vi "Rectangular Target - 2013.vi"() -> ()   [LabVIEW 2012]
doc: "This VI demonstrates how to do target processing on a laptop computer. It uses the same MJPG VI as the dashboard, sets a few of the important camera properties that impact processing, and carries out the same processing steps as the RT example also included in this project."
uses:
  <vilib>/Rock Robotics/WPI/Camera/WPI_CameraImageSize.ctl
  <vilib>/Rock Robotics/WPI/Camera/WPI_CameraWhite Balance Values.ctl
  <vilib>/vision/NI_Vision_Development_Module.lvlib
panel:
  in  "Camera Type":enum16{"206", "1011"}(ring)=enum."1011"
  in  "Image Source":enum32{"File Images", "Live Camera"}(tab)
  in  "Directory":path
  in  "File List":i32(listbox)
  in  "Camera IP Address":string="192.168.0.90"
  in  "Camera Settings":T2={"FPS"=30, "Compression"=30, "Image Size"=enum."320x240"}
  out "Target Info":T3(array[cluster])
  in  "Area Size Limit %":dbl=0.5
  in  "Particle Count Limit":i32=10
  in  "Score Limits":T4={"Rect Coverage"=60.0, "X Edge Strength"=40.0, "Y Edge Strength"=60.0, "Center"=75.0, "Outer"=75.0}
  in  "Processing":enum32{"Color", "Monochrome"}(tab)
  out "Value":cluster{i32, i32}
  out "Saturation":cluster{i32, i32}
  in  "Value":i32=255
  in  "Saturation":i32=255
  in  "Hue":i32(knob)=65 scale=0.0..255.0
  in  "Margins":cluster{"Hue":i32, "Sat":i32, "Val":i32}={"Hue"=33, "Sat"=53, "Val"=9} {"Sat" scale=0.0..80.0; "Val" scale=0.0..80.0; "Hue" scale=0.0..80.0}
  out "Hue":cluster{i32, i32}
  in  "Range":cluster{"Lower value":sgl, "Upper value":sgl}={"Lower value"=150.0, "Upper value"=255.0} {"Lower value" scale=0.0..255.0; "Upper value" scale=0.0..255.0}
  in  "Color Plane":i32(ring)=6 items=["Red", "Green", "Blue", "Hue", "Saturation", "Luminance", "Value", "Intensity"]
  in  "Annotate":bool=TRUE
  out "Processed Image":T5(plugin-control)
  out "Original Image":T5(plugin-control)
  # "Information:\nProcessing can be based on color or light intensity.\nParticles within the image are scored by rectangle coverage, aspect ratio, and\nedge strength/hollowness. A particle is considered a target if all scores\nare above the score limits you set. Particles can be annotated -- surrounded by\na rectangle and scores drawn to the left .\nTo control the number of particles being scored, use the count limit and the size\nlimit.\nBe sure to set the Camera IP before running. The distance calculation uses the\ncamera type to index the value of the lens view angle."
  # "Click in the image to choose  color for processing."
  # "Green scores are above the limit, orange are below. Inner/outer rect\nindicates all passed."
  # "Set before running."
  # "Lower/Upper"
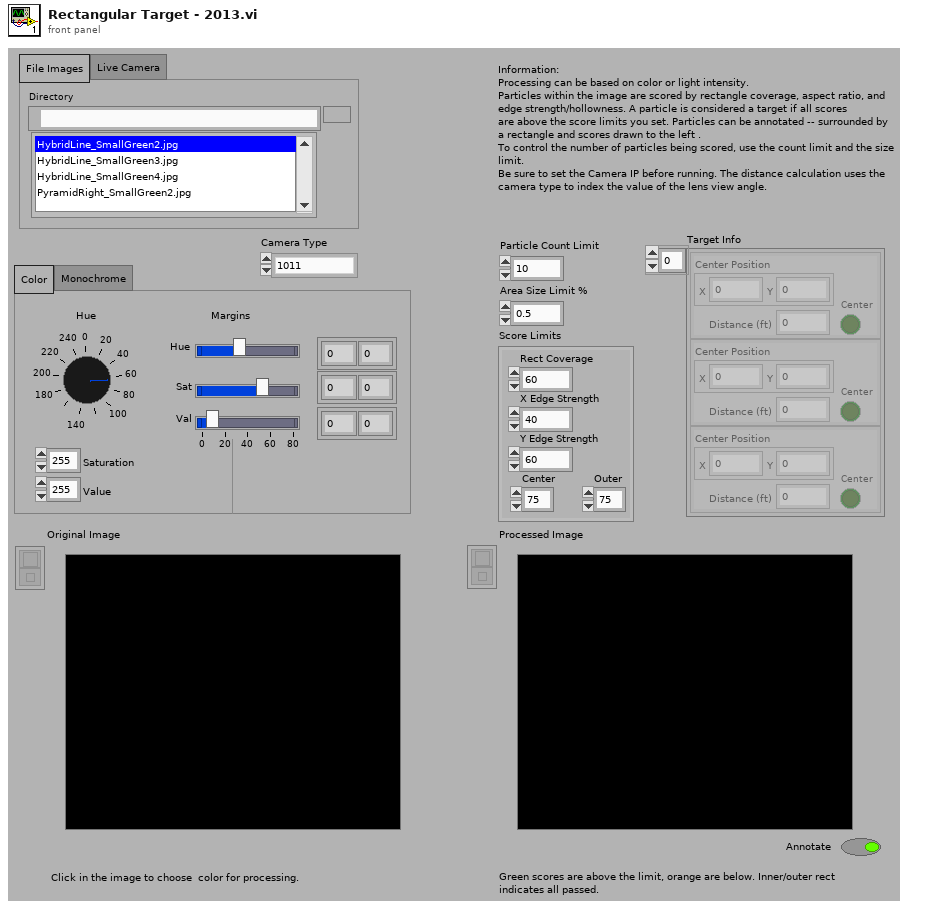
[diagram p1: front panel]
types:
  T1 = typedef "WPI_CameraImageSize.ctl" = enum16{"640x480", "320x240", "160x120"}
  T2 = cluster{"FPS":i32, "Compression":i32, "Image Size":T1}
  T3 = cluster{"Center Position":cluster{"X":dbl, "Y":dbl}, "Distance (ft)":dbl, "Center":bool}[]
  T4 = cluster{"Rect Coverage":dbl, "X Edge Strength":dbl, "Y Edge Strength":dbl, "Center":dbl, "Outer":dbl}
  T5 = typedef "IMAQ Image.ctl" = refnum<image>
  T6 = typedef "WPI_CameraWhite Balance Values.ctl" = enum16{"Auto", "Fixed indoor", "Fixed outdoor 1", "Fixed outdoor 2", "Fixed fluorescent 1", "Fixed fluorescent 2", "Hold current"}
  T7 = typedef "Image Type" = u32
  T8 = typedef "WPI_CameraDevRef.ctl" = cluster{"Camera Address":string, "CameraStatus":errorcluster, "Acquire Image Notifier":refnum<notifier>}
  T9 = cluster{"Position":cluster{"X":dbl, "Y":dbl}, "Distance (ft)":dbl, bool}[]
  T10 = cluster{cluster{"Left":dbl, "Top":dbl, "Right":dbl, "Bottom":dbl}, "Scores":dbl[], cluster{"Long":dbl, "Short":dbl}}[]
  T11 = cluster{"Target Center (-1 to 1)":cluster{"X":dbl, "Y":dbl}, "Distance (ft)":dbl, "Center Target":bool}
  T12 = cluster{"Target Center (-1 to 1)":cluster{"X":dbl, "Y":dbl}, "Distance (ft)":dbl, "Center Target":bool}[]
  T13 = cluster{"Left":dbl, "Top":dbl, "Right":dbl, "Bottom":dbl}
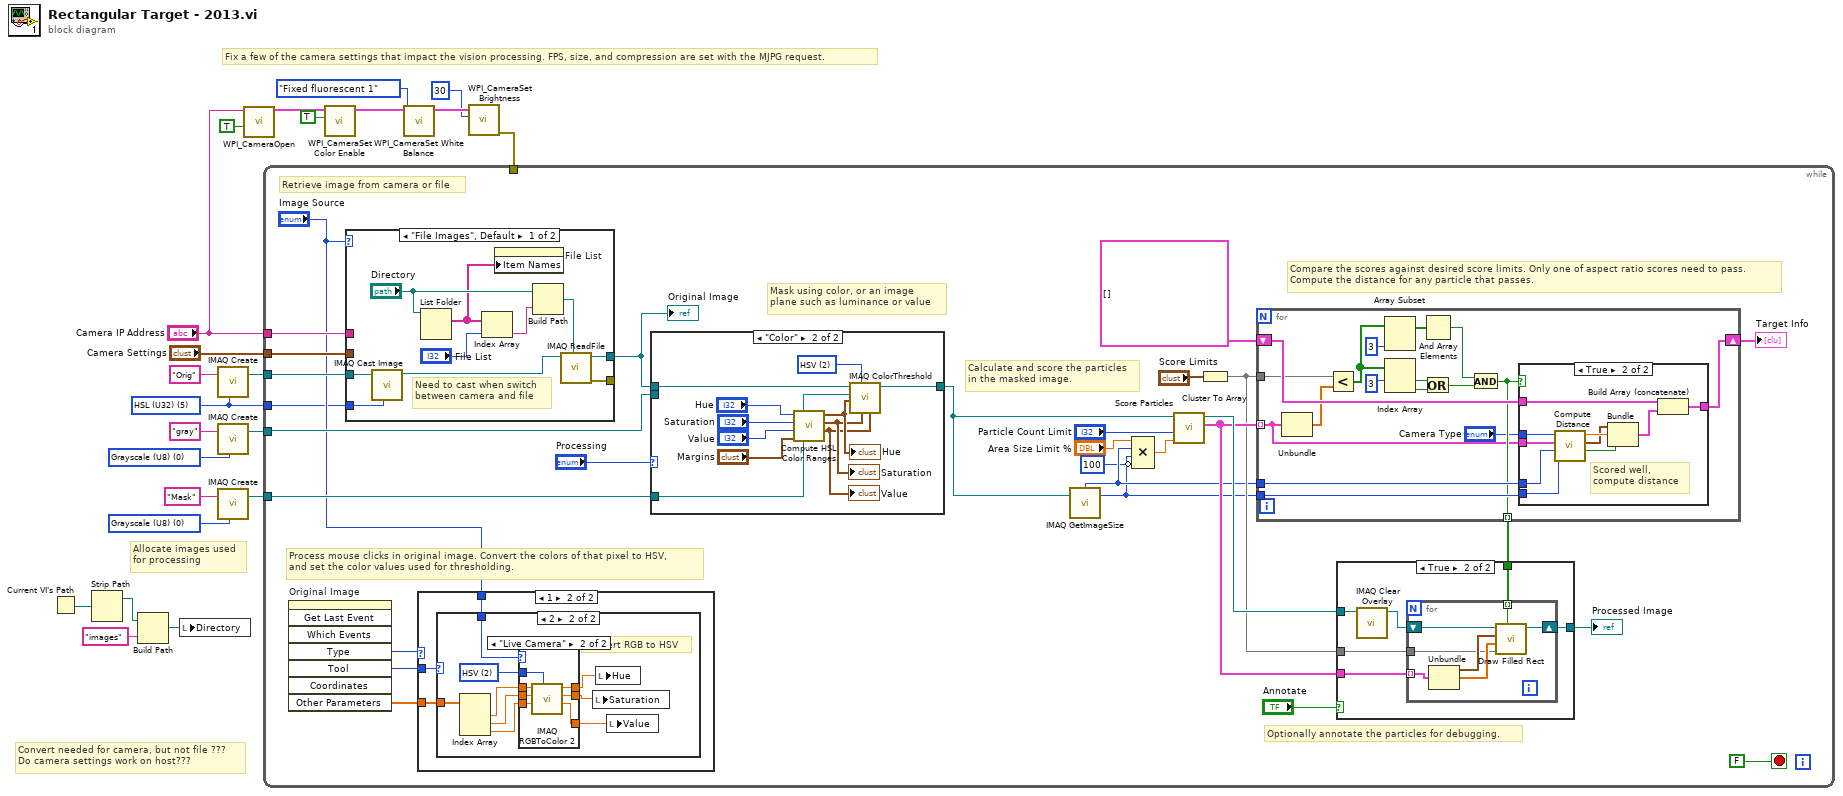
[diagram p0: block diagram]
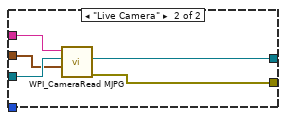
[diagram p2: hidden frame]
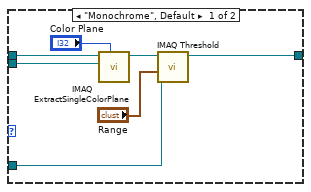
[diagram p4: hidden frame]
diagram:
  w17 = T7 0 items=["Grayscale (U8)", "Grayscale (I16)", "Grayscale (SGL)", "Complex (CSG)", "RGB (U32)", "HSL (U32)", "RGB (U64)", "Grayscale (U16)"] ("Image Type")
  w1 = T7 5 items=["Grayscale (U8)", "Grayscale (I16)", "Grayscale (SGL)", "Complex (CSG)", "RGB (U32)", "HSL (U32)", "RGB (U64)", "Grayscale (U16)"] ("Image Type")
  w23 = T7 0 items=["Grayscale (U8)", "Grayscale (I16)", "Grayscale (SGL)", "Complex (CSG)", "RGB (U32)", "HSL (U32)", "RGB (U64)", "Grayscale (U16)"] ("Image Type")
  # "Convert needed for camera, but not file ???\nDo camera settings work on host???"
  # "Allocate images used\nfor processing"
  # "Fix a few of the camera settings that impact the vision processing. FPS, size, and compression are set with the MJPG request."
  n1 = Current VI's Path() -> (path=w5:path)
  n2 = Strip Path(path=w5) -> (stripped path=w3:path)  [unwired: 1 out]
  n3 = Build Path(base path=w3, name or relative path="images") -> (appended path=w2:path)
  n4 = local write "Directory"(w2) -> ()
  n5 = call "IMAQ Create"("Image Name"="Orig", "Image Type"=w1) -> ("New Image"=w20:T5)  [unwired: 2 in, 2 out]
  n6 = call "IMAQ Create"("Image Name"="gray", "Image Type"=w23) -> ("New Image"=w19:T5)  [unwired: 2 in, 2 out]
  n7 = call "IMAQ Create"("Image Name"="Mask", "Image Type"=w17) -> ("New Image"=w16:T5)  [unwired: 2 in, 2 out]
  n8 = call <vilib>:"WPI_CameraOpen.vi"("Disallow Simulation"=TRUE, "Camera Address"="Camera IP Address") -> ("CameraDevRef"=w12:T8)  [unwired: 8 in, 1 out]
  n9 = call <vilib>:"WPI_CameraSet Color Enable.vi"("Color Enabled"=TRUE, "CameraDevRef"=w12) -> ("CameraDevRef Out"=w10:T8)  [unwired: 8 in, 1 out]
  n10 = call <vilib>:"WPI_CameraSet White Balance.vi"("White Balance"=WPI_CameraWhite_Balance_Values."Fixed fluorescent 1", "CameraDevRef"=w10) -> ("CameraDevRef Out"=w8:T8)  [unwired: 8 in, 1 out]
  n11 = call <vilib>:"WPI_CameraSet Brightness.vi"("Brightness"=30, "CameraDevRef"=w8) -> ("error out"=w14:errorcluster)  [unwired: 8 in, 1 out]
  n12 = while {
    tunnel: w20 -> [w45]
    tunnel: w19 -> [w52]
    tunnel: w16 -> [w31]
    tunnel: "Camera IP Address" -> [w43]
    tunnel: w14 -> [_]
    tunnel: "Camera Settings" -> [w34]
    tunnel: w1 -> [w29]
    stop <- FALSE stop-if-true
    # "Retrieve image from camera or file"
    # "Optionally annotate the particles for debugging."
    # "Compare the scores against desired score limits. Only one of aspect ratio scores need to pass.\nCompute the distance for any particle that passes."
    # "Process mouse clicks in original image. Convert the colors of that pixel to HSV,\nand set the color values used for thresholding."
    # "Calculate and score the particles\nin the masked image."
    # "Mask using color, or an image\nplane such as luminance or value"
    n13 = invoke on="Original Image" class="ImageControl" method="Get Last Event"() -> ("Type"=w46:i32, "Tool"=w47:i32, "Other Parameters"=w48:sgl[])  [unwired: 8 in, 5 out]
    n14 = case shown="\"File Images\", Default" "Image Source" {
      tunnel: w45 -> [w55 w67]
      tunnel: [w62 w66] -> w44
      tunnel: w43 -> [_ w65]
      tunnel: w34 -> [_ w64]
      tunnel: [w61 w63] -> _
      tunnel: w29 -> [w53 _]
      frame "File Images", Default {
        # "Need to cast when switch\nbetween camera and file"
        n15 = call "IMAQ Cast Image"("Image Type"=w53, "Image Src"=w55) -> ("Image Dst Out"=w54:T5)  [unwired: 8 in, 1 out]
        n16 = List Folder(path="Directory") -> (filenames=w56:string[])  [unwired: 3 in, 3 out]
        n17 = Index Array(array=w56, index="File List") -> (element=w59:string)
        n18 = property on="File List" class="LstBox (strict)"("Item Names"=w56) -> ()  [unwired: 2 in, 2 out]
        n19 = Build Path(base path="Directory", name or relative path=w59) -> (appended path=w58:path)
        n20 = call "IMAQ ReadFile"("File Path"=w58, "Image"=w54) -> ("error out"=w61:errorcluster, "Image Out"=w62:T5)  [unwired: 5 in, 3 out]
      }
      frame "Live Camera" {
        n21 = call <vilib>:"WPI_CameraRead MJPG.vi"("Camera Settings"=w64, "Image"=w67, "address"=w65) -> ("error out"=w63:errorcluster, "Image Out"=w66:T5)  [unwired: 6 in, 1 out]
      }
    }
    "Original Image" <- w44
    n22 = case shown="1" w46 {
      tunnel: w47 -> [_ w130]
      tunnel: w48 -> [_ w129]
      tunnel: "Image Source" -> [_ w128]
      frame 0, Default {
      }
      frame 1 {
        n23 = case shown="2" w130 {
          tunnel: w129 -> [_ w139]
          tunnel: w128 -> [_ w131]
          frame Default {
          }
          frame 2 {
            w138 = u16 2 items=["RGB", "HSL", "HSV", "HSI", "CIE L*a*b*", "CIE XYZ"] ("Color Mode")
            # "Convert RGB to HSV"
            n24 = Index Array(array=w139) -> (element #1=w137:sgl, element #2=w135:sgl, element #3=w133:sgl)  [unwired: 3 in]
            n25 = case shown="\"Live Camera\"" w131 {
              tunnel: w138 -> [_ w149]
              tunnel: w137 -> [w142 w148]
              tunnel: [w142 w147] -> w136
              tunnel: w135 -> [w141 w146]
              tunnel: [w141 w145] -> w134
              tunnel: w133 -> [w140 w144]
              tunnel: [w140 w143] -> w132
              frame "File Images", Default {
              }
              frame "Live Camera" {
                n26 = call "IMAQ RGBToColor 2"("Color Mode"=w149, "Blue value"=w144, "Green value"=w146, "Red value"=w148) -> ("Blue or Luma or Val or Inten or Z or b*value"=w143:dbl, "Green or Sat or Y or a* value"=w145:dbl, "Red or Hue or X or L* value"=w147:dbl)  [unwired: 4 in, 1 out]
              }
            }
            n27 = local write "Saturation"(w134) -> ()
            n28 = local write "Hue"(w136) -> ()
            n29 = local write "Value"(w132) -> ()
          }
        }
      }
    }
    n30 = case shown="\"Color\"" "Processing" {
      tunnel: w44 -> [w88 w99]
      tunnel: w52 -> [w87 _]
      tunnel: [w84 w98] -> w37
      tunnel: w31 -> [w82 w89]
      frame "Monochrome", Default {
        n31 = call "IMAQ ExtractSingleColorPlane"("Color Plane"="Color Plane", "Image Dst"=w87, "Image Src"=w88) -> ("Image Dst Out"=w86:T5)  [unwired: 1 in, 7 out]
        n32 = call "IMAQ Threshold"("Range"="Range", "Image Dst"=w82, "Image Src"=w86) -> ("Image Dst Out"=w84:T5)  [unwired: 3 in, 5 out]
      }
      frame "Color" {
        w97 = u16 2 items=["RGB", "HSL", "HSV", "HSI"] ("Color Mode")
        n33 = call "Compute HSL Color Ranges.vi"("Margins"="Margins", "Luminance"="Value", "Saturation"="Saturation", "Hue"="Hue") -> ("Lum Range"=w90:cluster{i32, i32}, "Sat Range"=w91:cluster{i32, i32}, "Hue Range"=w96:cluster{i32, i32})  [unwired: 5 in]
        "Hue" <- w96
        "Saturation" <- w91
        "Value" <- w90
        n34 = call "IMAQ ColorThreshold"("Blue or Luma or Val or Inten Range"=w90, "Green or Sat Range"=w91, "Color Mode"=w97, "Red or Hue Range"=w96, "Image Dst"=w89, "Image Src"=w99) -> ("Image Dst Out"=w98:T5)  [unwired: 4 in, 1 out]
      }
    }
    n35 = call "IMAQ GetImageSize"("Image"=w37) -> ("Y Resolution"=w26:i32, "X Resolution"=w27:i32)  [unwired: 3 in, 1 out]
    n36 = Compound Arithmetic op=MULTIPLY("Area Size Limit %", w27, w26, invert 100 ("value")) -> (w25:dbl)
    n37 = call "Score Particles.vi"("Area Size Limit"=w25, "Particle Count Limit"="Particle Count Limit", "Image Refnum in"=w37) -> ("Scored Particle Info"=w39:T10, "Image Refnum out"=w42:T5)  [unwired: 7 in]
    n38 = Cluster To Array(cluster="Score Limits") -> (array=w33:dbl[])
    n39 = for {
      shift-right: [w115] -> w49
      shift-left: T9 [] -> [w116]
      tunnel: w27 -> [w114]
      tunnel: w39 -> [w100] mode=indexing
      tunnel: w33 -> [w112]
      tunnel: w26 -> [w111]
      tunnel: [w102] -> w32 mode=indexing
      n40 = Unbundle(w100) -> ("Scores"=w113:dbl[])  [unwired: 2 out]
      n41 = Less?(x=w112, y=w113) -> (x < y?=w108:bool[])
      n42 = Array Subset(array=w108, length=3) -> (w109:bool[])  [unwired: 1 in]
      n43 = Index Array(array=w108, index #1=3 ("length")) -> (element #1=w106:bool, element #2=w105:bool)  [unwired: 1 in]
      n44 = And Array Elements(Boolean array=w109) -> (logical AND=w103:bool)
      n45 = Or(x=w106, y=w105) -> (x .or. y?=w104:bool)
      n46 = And(x=w103, y=w104) -> (x .and. y?=w102:bool)
      n47 = case shown="True" w102 {
        tunnel: w116 -> [w117 w127]
        tunnel: [w117 w126] -> w115
        tunnel: w114 -> [_ w124]
        tunnel: "Camera Type" -> [_ w122]
        tunnel: w111 -> [_ w120]
        tunnel: w100 -> [_ w119]
        frame False {
          # "Didn't score well enough"
        }
        frame True {
          # "Scored well,\ncompute distance"
          n48 = call "Compute Distance.vi"("Y Image Resolution"=w120, "X Image Resolution"=w124, "Particle Scores"=w119, "Camera Type"=w122) -> ("Center Target"=w118:bool, "Target Center (-1 to 1)"=w121:cluster{"X":dbl, "Y":dbl}, "Distance (ft)"=w123:dbl)  [unwired: 5 in]
          n49 = Bundle("Target Center (-1 to 1)"=w121, "Distance (ft)"=w123, "Center Target"=w118) -> (w125:T11)  [unwired: 1 in]
          n50 = Build Array (concatenate)(w127, w125) -> (w126:T12)
        }
      }
    }
    "Target Info" <- w49
    n51 = case shown="True" "Annotate" {
      tunnel: w42 -> [w68 w74]
      tunnel: [w68 w73] -> w40
      tunnel: w39 -> [_ w71]
      tunnel: w33 -> [_ w70]
      tunnel: w32 -> [_ w69]
      frame False {
      }
      frame True {
        n52 = call "IMAQ Clear Overlay"("Image"=w74) -> ("Image Out"=w72:T5)  [unwired: 2 in, 8 out]
        n53 = for {
          shift-right: [w80] -> w73
          shift-left: w72 -> [w81]
          tunnel: w71 -> [w77] mode=indexing
          tunnel: w70 -> [w76]
          tunnel: w69 -> [w75] mode=indexing
          n54 = Unbundle(w77) -> (w78:T13, "Scores"=w79:dbl[])  [unwired: 1 out]
          n55 = call "Draw Filled Rect.vi"("Limit Passed"=w75, "Limits"=w76, "Scores"=w79, "Bounding Box"=w78, "image in"=w81) -> ("image out"=w80:T5)  [unwired: 6 in]
        }
      }
    }
    "Processed Image" <- w40
  }
